vi "Read ref.vi"(8 "error in (no error)":errorcluster, 11 "Generic In":refnum<class "Generic.lvclass">) -> (0 "error out":errorcluster, 2 "ref":refnum<vi>, 3 "Generic Out":refnum<class "Generic.lvclass">)   [LabVIEW 2023, in "TLC_Scripto.lvlib" / "Generic.lvclass"]
uses:
  Generic.lvclass
  Generic.lvclass/Generic.ctl
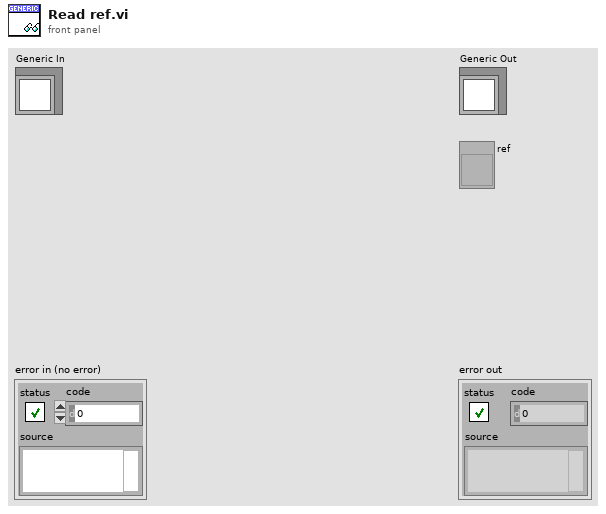
[diagram p1: front panel]
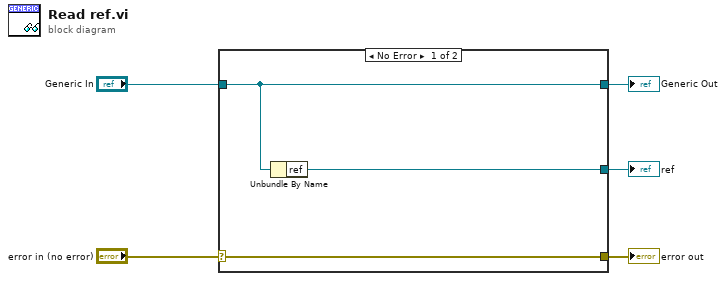
[diagram p0: block diagram]
diagram:
  n1 = case shown="No Error" "error in (no error)" {
    selector: "error in (no error)" -> [w8 w9]
    tunnel: [w8 w9] -> w4
    tunnel: [w7 w10] -> w2
    tunnel: "Generic In" -> [w7 w10]
    tunnel: [w6 _] -> w1
    frame No Error {
      n2 = Unbundle By Name(w7) -> ("ref"=w6:refnum<vi>)
    }
    frame Error {
    }
  }
  "error out" <- w4
  "Generic Out" <- w2
  "ref" <- w1
